vi "NI 9213 Getting Started (Host) Chas2.vi"(5 "RIO Device":T4="RIO0::INSTR") -> ()   [LabVIEW 2011]
doc: "This VI runs on the host device. The host can be a Windows PC or Real-Time target. The example downloads and runs an FPGA VI that continuously reads single point values from all 16 channels of a NI 9213 module."
uses:
  <vilib>/userDefined/High Color/nirio_resource_hc.ctl
  Program Files (x86)/National Instruments/LabVIEW 2011/examples/CompactRIO/Shared/cRIO Convert Thermocouple Readings.llb/Thermocouple Type.ctl
  <vilib>/LabVIEW Targets/FPGA/cRIO/shared/nicrio_ModuleControls/nicrio_BasicConversionTime.ctl
  <vilib>/FPGAPlugInAG/cRIO-9074/niLvFpga_Open_cRIO-9074.vi
  <vilib>/rvi/interface/common/dynamic/niFpgaDynamicAddResources.vi
  <vilib>/FPGAPlugInAG/Dynamic/niLvFpga_Run_Dynamic.vi
  <vilib>/Utility/error.llb/Error Cluster From Error Code.vi
  <vilib>/rvi/errors/niLvFpgaAdjustHostInterfaceError.vi
  Program Files (x86)/National Instruments/LabVIEW 2011/examples/CompactRIO/Module Specific/NI 9213/NI 9213 Support Files.llb/NI 9213 Convert to Temperature (Calibrated).vi
  <vilib>/FPGAPlugInAG/Dynamic/niLvFpga_Close_Dynamic.vi
  <vilib>/rvi/interface/nirviOpenFPGA/nirviOpenFPGA.xnode
  FPGA Bitfiles/MAXCATTestProjec_FPGATarget2_NI9213GettingSta_497D52F4.lvbitx
  NI 9213 Getting Started (FPGA) Chas2.vi
  <vilib>/rvi/interface/nirviMethod/nirviMethod.xnode
  <vilib>/rvi/interface/nirviReadWriteControl/nirviReadWriteControl.xnode
  <vilib>/rvi/interface/nirviCloseFPGA/nirviCloseFPGA.xnode
  <vilib>/rvi/interface/nirviMethod/StockFPGA_InlinedMethodWaitForSingleIRQ.vi
  <vilib>/FPGAPlugInAG/Dynamic/niLvFpga_WaitOnIrq_Dynamic.vi
  NiFpgaLv.dll
  <vilib>/rvi/interface/Simulation/niFpgaSimulationCallBeginRW.vi
  <vilib>/FPGAPlugInAG/Dynamic/niLvFpga_AcknowledgeIrq_Dynamic.vi
panel:
  in  "Conversion Time":T1=enum."High Resolution"
  in  "Update":bool
  in  "ThermocoupleType":T2=2 items=["B", "E", "J", "K", "R", "S", "T", "N"]
  out "TC Status":T3
  out "Thermocouple Temperature":T5(graph)
  in  "stop":bool
  # "For instructions, select  Help>>Show Context Help and hover over the icon."
  # "Resource Parameters"
  # "Timing Parameters"
  # "Thermocouple  Parameters"
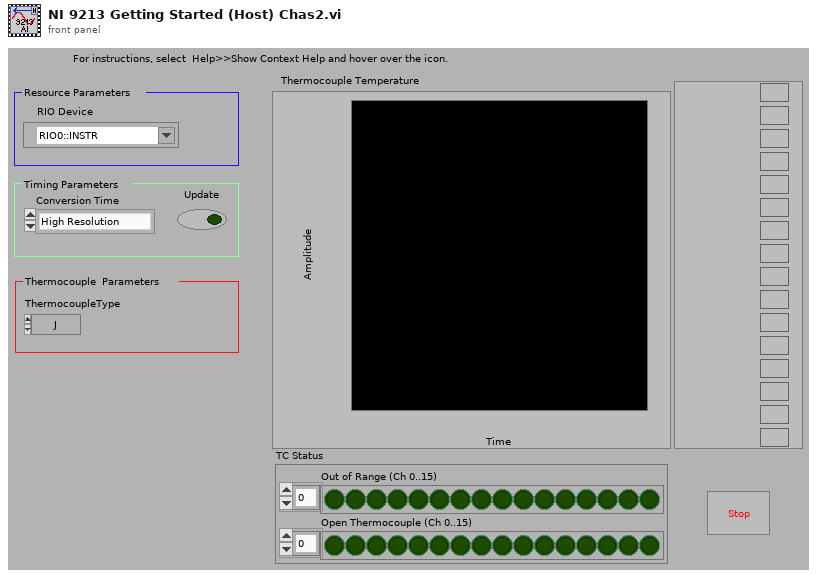
[diagram p1: front panel]
types:
  T1 = typedef "nicrio_BasicConversionTime.ctl" = enum8{"High Speed", "High Resolution"}
  T2 = typedef "Thermocouple Type.ctl" = u16
  T3 = cluster{"Out of Range (Ch 0..15)":bool[], "Open Thermocouple (Ch 0..15)":bool[]}
  T4 = typedef "nirio_resource_hc.ctl" = tag
  T5 = cluster{"[0]":dbl, "[1]":dbl, "[2]":dbl, "[3]":dbl, "[4]":dbl, "[5]":dbl, "[6]":dbl, "[7]":dbl, "[8]":dbl, "[9]":dbl, "[10]":dbl, "[11]":dbl, "[12]":dbl, "[13]":dbl, "[14]":dbl, "[15]":dbl}
  T6 = cluster{"Mod1/TC0":fxp<+/-,24,-2>, "Mod1/TC1":fxp<+/-,24,-2>, "Mod1/TC2":fxp<+/-,24,-2>, "Mod1/TC3":fxp<+/-,24,-2>, "Mod1/TC4":fxp<+/-,24,-2>, "Mod1/TC5":fxp<+/-,24,-2>, "Mod1/TC6":fxp<+/-,24,-2>, "Mod1/TC7":fxp<+/-,24,-2>, "Mod1/TC8":fxp<+/-,24,-2>, "Mod1/TC9":fxp<+/-,24,-2>, "Mod1/TC10":fxp<+/-,24,-2>, "Mod1/TC11":fxp<+/-,24,-2>, "Mod1/TC12":fxp<+/-,24,-2>, "Mod1/TC13":fxp<+/-,24,-2>, "Mod1/TC14":fxp<+/-,24,-2>, "Mod1/TC15":fxp<+/-,24,-2>, "Mod1/AutoZero":fxp<+/-,24,-2>, "Mod1/CJC":fxp<+/-,24,-2>}
  T7 = cluster{"Out of Range":bool[], "Open Thermocouple":bool[]}
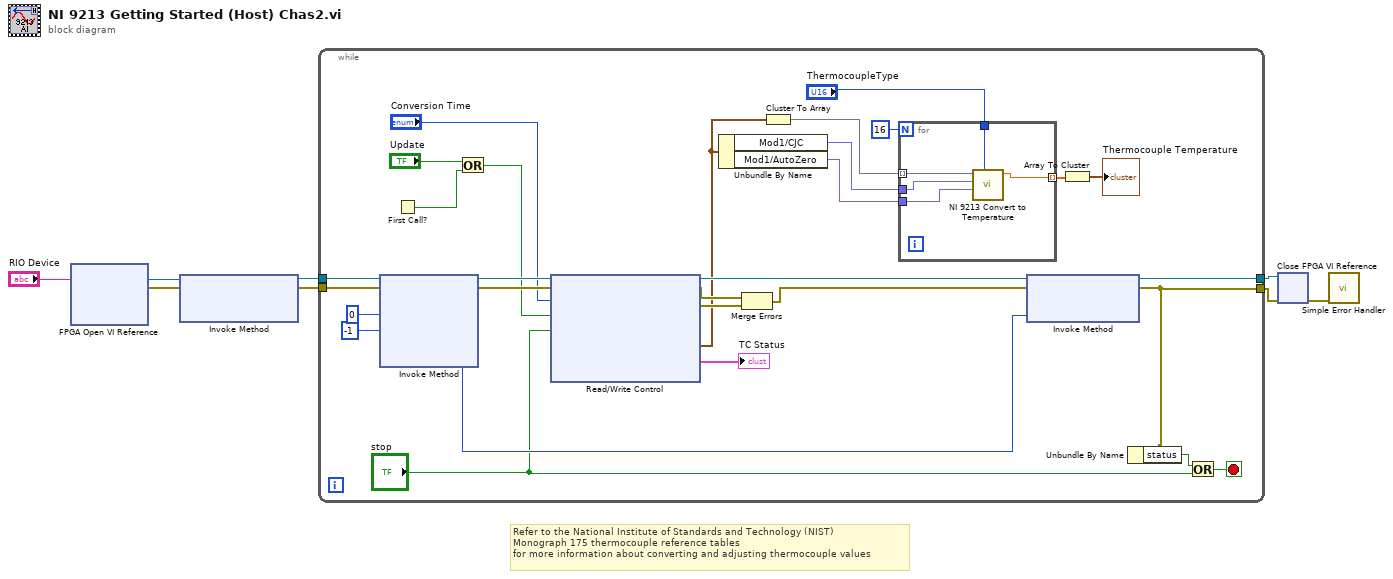
[diagram p0: block diagram]
diagram:
  # "Refer to the National Institute of Standards and Technology (NIST) \nMonograph 175 thermocouple reference tables \nfor more information about converting and adjusting thermocouple values"
  n1 = xnode "FPGA Open VI Reference"("resource name"="RIO Device") -> ("FPGA VI Reference Out"=w4:refnum<k20>, "error out"=w3:errorcluster)  [unwired: 1 in]
  n2 = xnode "Invoke Method"("FPGA VI Reference In"=w4, "error in"=w3) -> ("FPGA VI Reference Out"=w2:refnum<k20>, "error out"=w1:errorcluster)  [unwired: 1 in]
  n3 = while {
    tunnel: w2 -> [w37]
    tunnel: w1 -> [w36]
    tunnel: [w30] -> w8
    tunnel: [w27] -> w7
    stop <- w28 stop-if-true
    n4 = xnode "Invoke Method"("FPGA VI Reference In"=w37, "error in"=w36, "IRQ Number(s)"=0, "Timeout (ms)"=-1 ("timeout (ms)(-1 for no timeout)")) -> ("FPGA VI Reference Out"=w33:refnum<k20>, "error out"=w32:errorcluster, "IRQ(s) Asserted"=w29:i32)  [unwired: 1 out]
    n5 = First Call?() -> (First Call?: T/F=w11:bool)
    n6 = Or(x="Update", y=w11) -> (x .or. y?=w9:bool)
    n7 = xnode "Read/Write Control"("FPGA VI Reference In"=w33, "error in"=w32, "Conversion Time"="Conversion Time", "Update Conversion Time"=w9, "Stop"="stop") -> ("FPGA VI Reference Out"=w31:refnum<k20>, "error out"=w23:errorcluster, "TC Output"=w17:T6, "FPGA Error Out"=w22:errorcluster, "TC Status"=→"TC Status":T7)
    n8 = Unbundle By Name(w17) -> ("Mod1/CJC"=w20:fxp<+/-,24,-2>, "Mod1/AutoZero"=w19:fxp<+/-,24,-2>)
    n9 = Merge Errors(w23, w22) -> (w21:errorcluster)
    n10 = Cluster To Array(cluster=w17) -> (array=w16:fxp<+/-,24,-2>[])
    n11 = for {
      N: 16 -> [_]
      tunnel: w16 -> [w42] mode=indexing
      tunnel: "ThermocoupleType" -> [w41]
      tunnel: w20 -> [w40]
      tunnel: w19 -> [w39]
      tunnel: [w38] -> w18 mode=indexing
      n12 = call-poly "NI 9213 Convert to Temperature.vi"("ThermocoupleType"=w41, "AutoZero"=w39, "CJC"=w40, "TC Input"=w42) -> ("Thermocouple Temperature"=w38:dbl)  [unwired: 1 in, 6 out]
    }
    n13 = xnode "Invoke Method"("FPGA VI Reference In"=w31, "error in"=w21, "IRQ Number(s)"=w29) -> ("FPGA VI Reference Out"=w30:refnum<k20>, "error out"=w27:errorcluster)
    n14 = Array To Cluster(array=w18) -> (cluster=→"Thermocouple Temperature":T5)
    n15 = Unbundle By Name(w27) -> ("status"=w26:bool)
    n16 = Or(x=w26, y="stop") -> (x .or. y?=w28:bool)
  }
  n17 = xnode "Close FPGA VI Reference"("FPGA VI Reference In"=w8, "error in"=w7) -> ("error out"=w6:errorcluster)
  n18 = call <vilib>:"Simple Error Handler.vi"("error in (no error)"=w6) -> ()  [unwired: 1 in, 8 out]
